vi "CSV_WRITE_READ.vi"() -> ()   [LabVIEW 2020]
uses:
  <vilib>/Utility/sysdir.llb/System Directory Type.ctl
  <vilib>/Utility/file.llb/Read Delimited Spreadsheet (DBL).vi
  <vilib>/Utility/file.llb/Write Delimited Spreadsheet (DBL).vi
panel:
  out "all rows":dbl[][](array[numeric]) caption="모든 행"
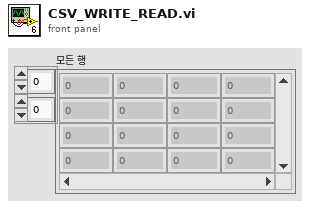
[diagram p1: front panel]
types:
  T1 = typedef "System Directory Type.ctl" = i32
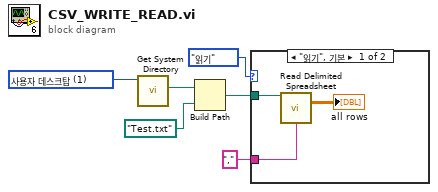
[diagram p0: block diagram]
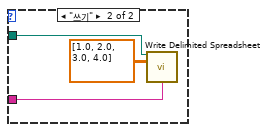
[diagram p2: hidden frame]
diagram:
  w6 = T1 1 items=["사용자 홈"=0, "사용자 데스크탑"=1, "사용자 문서"=2, "사용자 어플리케이션 데이터"=3, "사용자 환경"=4, "사용자 임시"=5, "퍼블릭 문서"=6, "퍼블릭 어플리케이션 데이터"=7, "퍼블릭 환경"=8, "퍼블릭 캐시"=13, "시스템 코어 라이브러리"=9, "시스템 설치된 라이브러리"=10, "어플리케이션 파일"=11, "부팅 볼륨 루트"=12] ("system directory type")
  n1 = call <vilib>:"Get System Directory.vi"("system directory type"=w6) -> ("system directory"=w4:path)  [unwired: 10 in]
  n2 = Build Path(base path=w4, name or relative path=path "Test.txt" ("이름 또는 상대 경로")) -> (appended path=w3:path)
  n3 = case shown="\"읽기\", 기본" enum16{"쓰기", "읽기", ""}."읽기" {
    tunnel: w3 -> [w9 w12]
    tunnel: "," ("delimiter (\\t)") -> [w8 w10]
    frame "읽기", Default {
      n4 = call-poly <vilib>:"Read Delimited Spreadsheet.vi"("file path (dialog if empty)"=w9, "delimiter (\\t)"=w8) -> ("all rows"=→"all rows":dbl[][])  [unwired: 8 in, 5 out]
    }
    frame "쓰기" {
      n5 = call-poly <vilib>:"Write Delimited Spreadsheet.vi"("file path (dialog if empty)"=w12, "2D data"=dbl[][] [[1.0, 2.0], [3.0, 4.0]], "delimiter (\\t)"=w10) -> ()  [unwired: 11 in, 2 out]
    }
  }
